vi "Host_Test.vi"() -> ()   [LabVIEW 2012]
uses:
  <vilib>/rvi/interface/nirviOpenFPGA/nirviOpenFPGA.xnode
  <vilib>/rvi/interface/nirviReadWriteControl/nirviReadWriteControl.xnode
  <vilib>/rvi/interface/Simulation/niFpgaSimulationCallBeginRW.vi
  <vilib>/rvi/errors/niLvFpgaAdjustHostInterfaceError.vi
  <vilib>/rvi/interface/nirviMethod/nirviMethod.xnode
  <vilib>/rvi/interface/nirviCloseFPGA/nirviCloseFPGA.xnode
  FPGA Bitfiles/AnalogIntegrator_NI5771_PXIe-7962R.lvbitx
  AnalogIntegrator_NI5771/FPGA VIs/AnalogIntegrator_NI5771.vi
  <vilib>/FPGAPlugInAG/Dynamic/niLvFpga_Close_Dynamic.vi
  <vilib>/FPGAPlugInAG/Dynamic/niLvFpga_ReadFifo_Dynamic.vi
  <vilib>/rvi/errors/niLvFpgaMergeErrorWithErrorCode.vi
panel:
  in  "Baseline16 Ch1":u16
  in  "Requested Pixels":u32
  out "Resonance Trigger":i32[][](graph)
  in  "Samples per pixel":u32
  out "error out":errorcluster
  out "InterloopFIFO Overflow":bool
  out "ToHostCh1FIFO Overflow":bool
  out "Configured?":bool
  out "IO Module\\AI Over Range":bool
  out "Ch1":i32[][](graph)
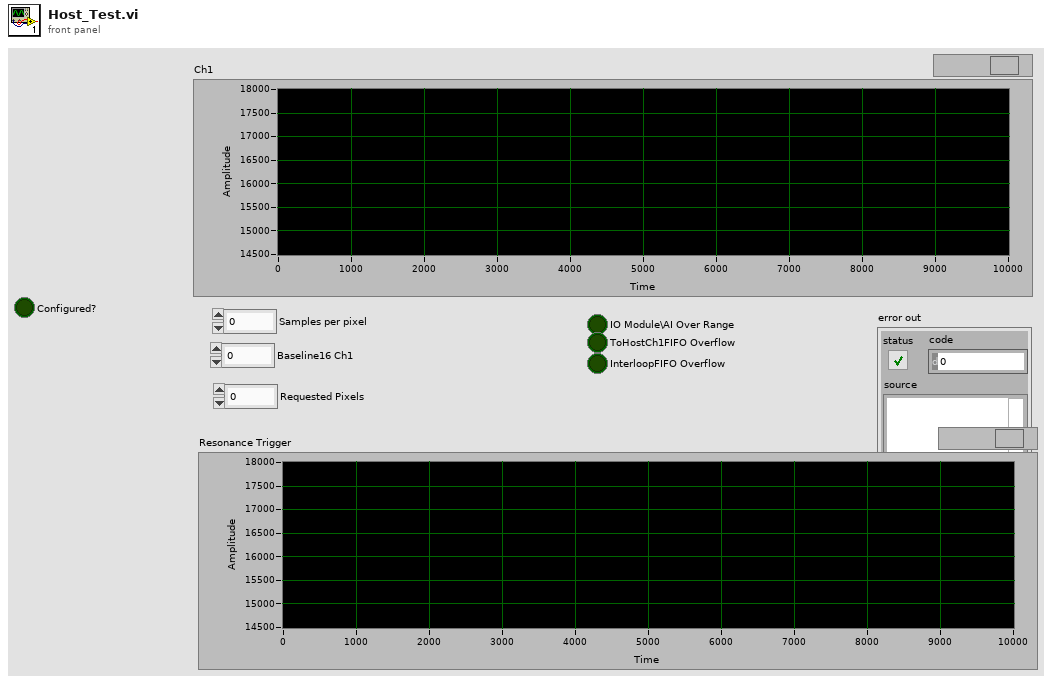
[diagram p1: front panel]
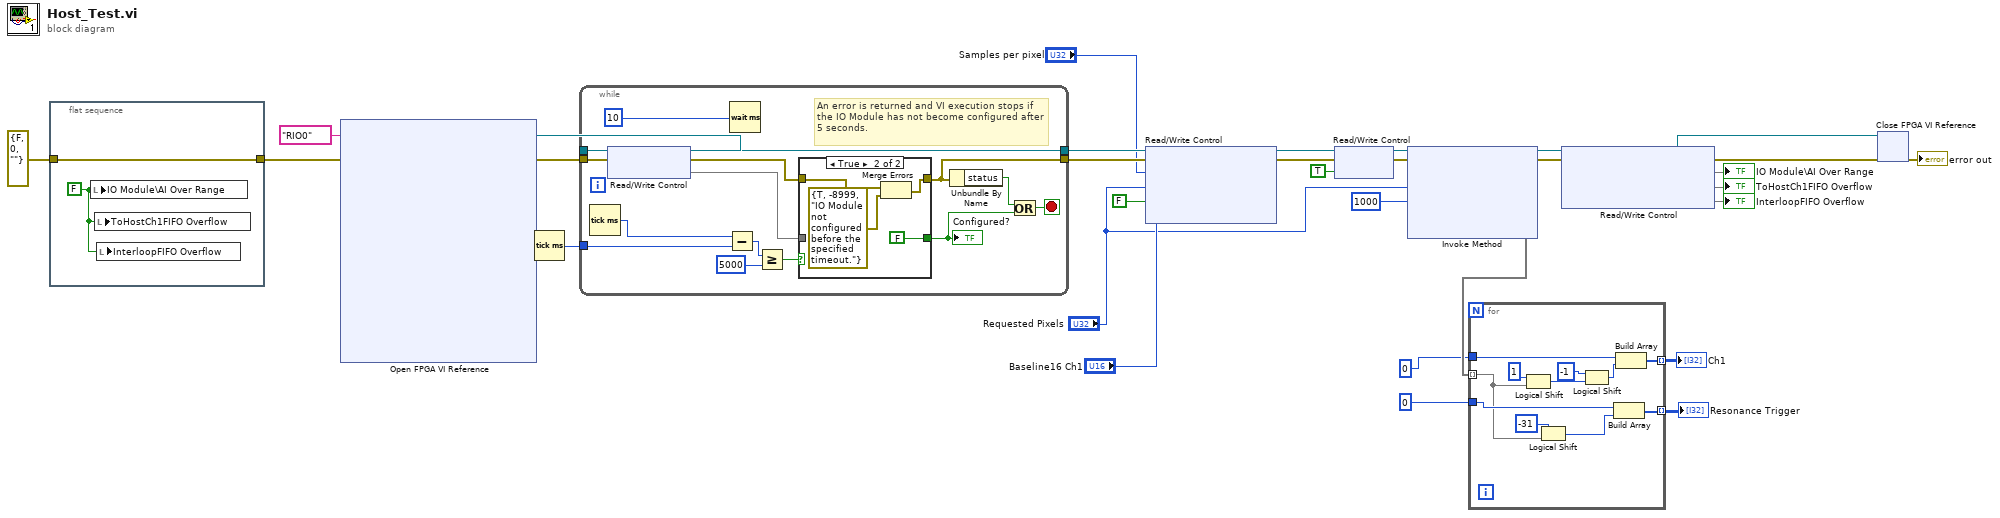
[diagram p0: block diagram]
diagram:
  n1 = flat-sequence {
    tunnel: errorcluster {"status"=FALSE, "code"=0, "source"=""} ("error in") -> [w32]
    tunnel: [w32] -> w10
    frame #0 {
      w33 = FALSE ("IO Module\\AI Over Range")
      n2 = local write "IO Module\\AI Over Range"(w33) -> ()
      n3 = local write "ToHostCh1FIFO Overflow"(w33) -> ()
      n4 = local write "InterloopFIFO Overflow"(w33) -> ()
    }
  }
  n5 = xnode "Open FPGA VI Reference"("error in"=w10, "resource name"=tag "RIO0") -> ("FPGA VI Reference Out"=w17:refnum<k20>, "error out"=w18:errorcluster)
  n6 = Tick Count (ms)() -> (millisecond timer value=w16:u32)
  n7 = while {
    tunnel: w18 -> [w41]
    tunnel: [w45] -> w15
    tunnel: [w37] -> w14
    tunnel: w17 -> [w40]
    tunnel: w16 -> [w35]
    stop <- w43 stop-if-true
    # "An error is returned and VI execution stops if the IO Module has not become configured after 5 seconds."
    n8 = Tick Count (ms)() -> (millisecond timer value=w36:u32)
    n9 = xnode "Read/Write Control"("FPGA VI Reference In"=w40, "error in"=w41) -> ("FPGA VI Reference Out"=w37:refnum<k20>, "error out"=w38:errorcluster, "Configured?"=w39)
    n10 = Subtract(x=w36, y=w35) -> (x-y=w34:u32)
    n11 = Wait (ms)(milliseconds to wait=u32 10) -> ()  [unwired: 1 out]
    n12 = Greater Or Equal?(x=w34, y=u32 5000) -> (x >= y?=w46:bool)
    n13 = case shown="True" w46 {
      tunnel: [w50 FALSE ("Configured?")] -> w42
      tunnel: w39 -> [w50 _]
      tunnel: [w49 w53] -> w45
      tunnel: w38 -> [w49 w51]
      frame False {
      }
      frame True {
        n14 = Merge Errors(w51, errorcluster {"status"=TRUE, "code"=-8999, "source"="IO Module not configured before the specified timeout."} ("error in")) -> (w53:errorcluster)
      }
    }
    "Configured?" <- w42
    n15 = Unbundle By Name(w45) -> ("status"=w44:bool)
    n16 = Or(x=w44, y=w42) -> (x .or. y?=w43:bool)
  }
  n17 = xnode "Read/Write Control"("FPGA VI Reference In"=w14, "error in"=w15, "Samples per pixel"="Samples per pixel", "Requested pixels"="Requested Pixels", "Acquire continuously"=FALSE, "Baselinex8 Ch1"="Baseline16 Ch1") -> ("FPGA VI Reference Out"=w28:refnum<k20>, "error out"=w29:errorcluster)
  n18 = xnode "Read/Write Control"("FPGA VI Reference In"=w28, "error in"=w29, "Acquire"=TRUE) -> ("FPGA VI Reference Out"=w26:refnum<k20>, "error out"=w25:errorcluster)
  n19 = xnode "Invoke Method"("FPGA VI Reference In"=w26, "error in"=w25, "Number of Elements"="Requested Pixels", "Timeout (ms)"=1000) -> ("FPGA VI Reference Out"=w23:refnum<k20>, "error out"=w21:errorcluster, "Data"=w5:void[])  [unwired: 1 out]
  n20 = for {
    tunnel: w5 -> [w55] mode=indexing
    tunnel: 0 -> [w65]
    tunnel: 0 -> [w64]
    tunnel: [w63] -> w1 mode=indexing
    tunnel: [w62] -> w2 mode=indexing
    n21 = Logical Shift(y=i16 1, x=w55) -> (x << y=w57:i16)
    n22 = Logical Shift(y=i16 -31, x=w55) -> (x << y=w60:i16)
    n23 = Logical Shift(y=i16 -1, x=w57) -> (x << y=w56:i16)
    n24 = Build Array(w64, w60) -> (w63:i32[])
    n25 = Build Array(w65, w56) -> (w62:i32[])
  }
  "Ch1" <- w2
  "Resonance Trigger" <- w1
  n26 = xnode "Read/Write Control"("FPGA VI Reference In"=w23, "error in"=w21) -> ("FPGA VI Reference Out"=w22:refnum<k20>, "error out"=w20:errorcluster, "IO Module\\AI Over Range"=→"IO Module\\AI Over Range", "ToHostCh1FIFO Overflow"=→"ToHostCh1FIFO Overflow", "InterloopFIFO Overflow"=→"InterloopFIFO Overflow")
  n27 = xnode "Close FPGA VI Reference"("FPGA VI Reference In"=w22, "error in"=w20) -> ("error out"=→"error out":errorcluster)
